vi "SetArmTimer.vi"(8 "Error In":errorcluster, 10 "Interval (sec)":dbl=0.1 min=0.001 max=99999.99 step=0.001, 11 "Keithley 6482 In":refnum<visa-resource-name>) -> (0 "Error Out":errorcluster, 3 "Keithley 6482 Out":refnum<visa-resource-name>)   [LabVIEW 2014, in "Keithley-6482-Visa.lvlib"]
uses:
  Keithley-6482-Visa.lvlib
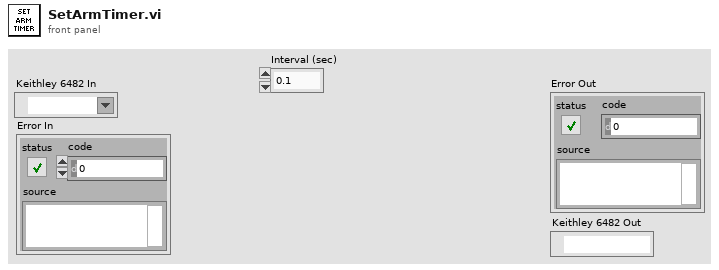
[diagram p1: front panel]
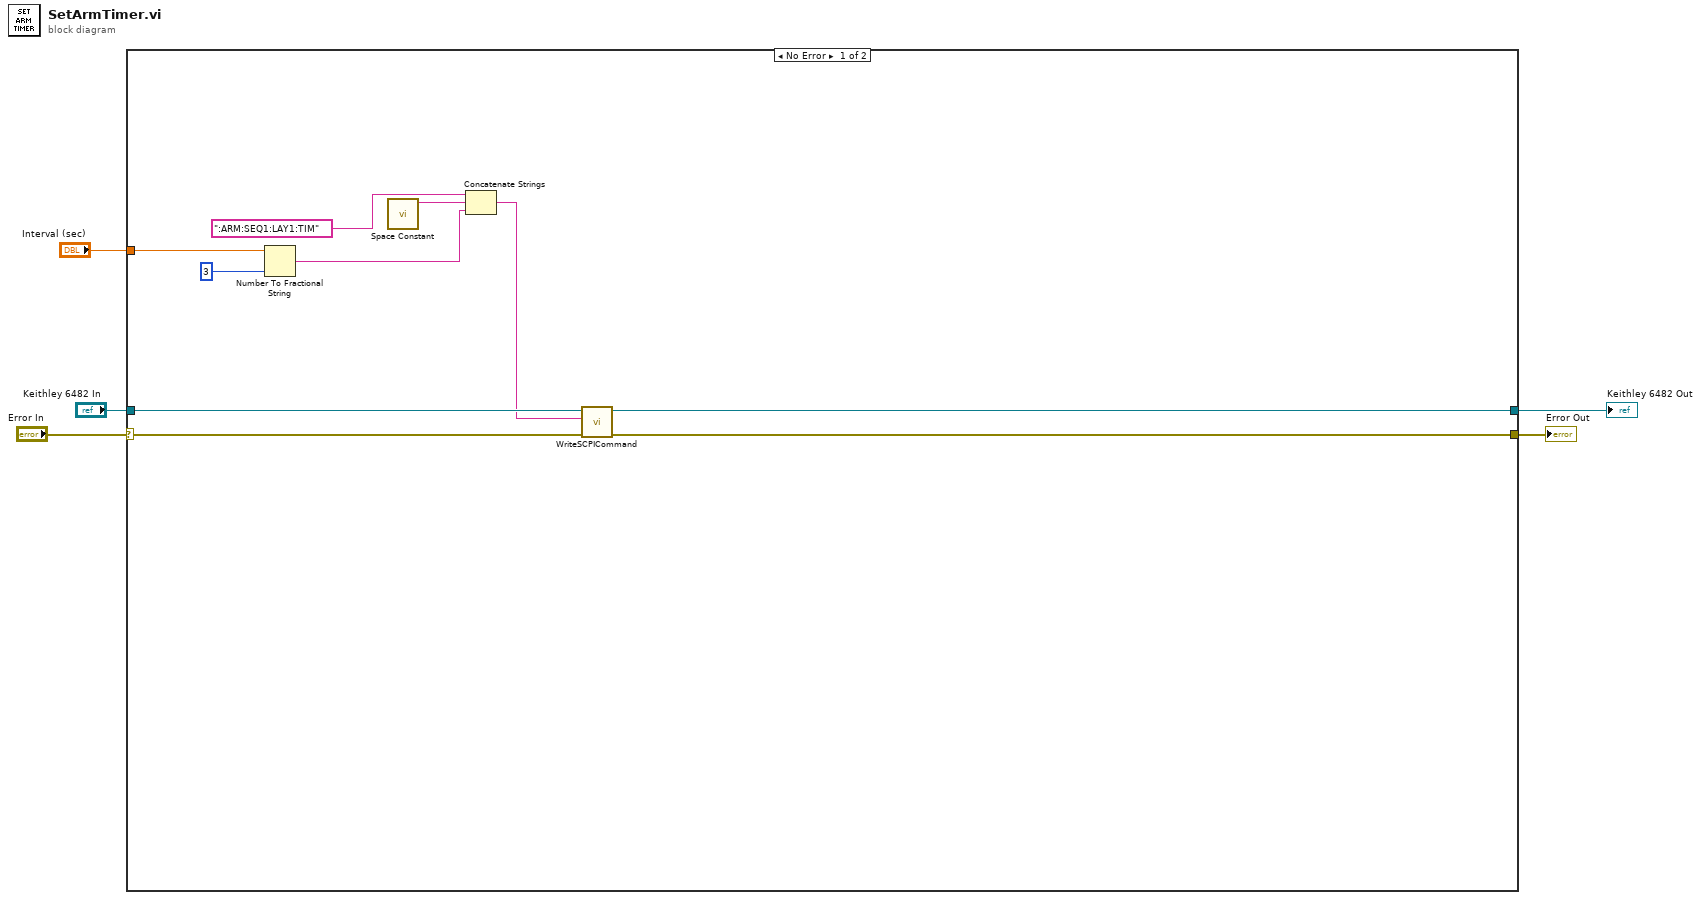
[diagram p0: block diagram]
diagram:
  n1 = case shown="No Error" "Error In" {
    selector: "Error In" -> [w15 w16]
    tunnel: "Keithley 6482 In" -> [w14 w17]
    tunnel: [w9 w16] -> w3
    tunnel: [w10 w17] -> w2
    tunnel: "Interval (sec)" -> [w8 _]
    frame No Error {
      n2 = Number To Fractional String(number=w8, precision (6)=i16 3) -> (F-format string=w6:string)  [unwired: 2 in]
      n3 = call <vilib>:"Space Constant.vi"() -> ("String"=w12:string)
      n4 = Concatenate Strings(":ARM:SEQ1:LAY1:TIM" ("string"), w12, w6) -> (w11:string)
      n5 = call "WriteSCPICommand.vi"("Error In"=w15, "SCPI Command"=w11, "Keithley 6482 In"=w14) -> ("Error Out"=w9:errorcluster, "Keithley 6482 Out"=w10:refnum<visa-resource-name>)  [unwired: 7 in]
    }
    frame Error {
    }
  }
  "Error Out" <- w3
  "Keithley 6482 Out" <- w2
